vi "DiffDrivePoseEst2_Execute.vi"(0 "Vision TImeStamp_Seconds":dbl=0.02, 3 "DiffPoseEst2Config":T1={"TrackWidth_Meters"=1.2, "Odom X std dev M"=0.02, "Odom Y std dev M"=0.02, "Odom Heading std dev Rad"=0.01, "Vision X std dev M"=0.1, "Vision Y std dev M"=0.1, "Vision Heading std dev Rad"=0.05} {"Vision Heading std dev Rad" format="%#_13g"; "Vision Y std dev M" format="%#_13g"; "Vision X std dev M" format="%#_13g"; "Odom Heading std dev Rad" format="%#_13g"; "Odom Y std dev M" format="%#_13g"; "Odom X std dev M" format="%#_13g"; "TrackWidth_Meters" format="%#_13g"}, 4 "visionRobotPose":T2={"TRANSLATION"={"X"=0.0, "Y"=0.0}, "ROTATION"={"VALUE"=0.0, "COS"=1.0, "SIN"=0.0}} {"ROTATION"."SIN" format="%13.4f"; "ROTATION"."COS" format="%13.4f"; "ROTATION"."VALUE" format="%13.4f"; "TRANSLATION"."Y" format="%14.3f"; "TRANSLATION"."X" format="%14.3f"}, 5 "Game Started":bool=TRUE, 6 "Add Vision Meas":bool, 7 "InitialPose":T2={"TRANSLATION"={"X"=0.0, "Y"=0.0}, "ROTATION"={"VALUE"=0.0, "COS"=1.0, "SIN"=0.0}} {"ROTATION"."SIN" format="%13.4f"; "ROTATION"."COS" format="%13.4f"; "ROTATION"."VALUE" format="%13.4f"; "TRANSLATION"."Y" format="%14.3f"; "TRANSLATION"."X" format="%14.3f"}, 8 "Pass Through Time":dbl=-1.0, 9 "Gyro Degrees":dbl, 10 "RightDistance_M":dbl=0.02, 11 "LeftDistance_M":dbl=0.02) -> (1 "Error":bool, 2 "Estimated Pose":T2={"TRANSLATION"={"X"=0.0, "Y"=0.0}, "ROTATION"={"VALUE"=0.0, "COS"=1.0, "SIN"=0.0}} {"ROTATION"."SIN" format="%13.4f"; "ROTATION"."COS" format="%13.4f"; "ROTATION"."VALUE" format="%13.4f"; "TRANSLATION"."Y" format="%14.3f"; "TRANSLATION"."X" format="%14.3f"})   [LabVIEW 2019, in "Trajectory_Library.lvlib"]
doc: "This single call LabVIEW function wraps Differential Drive Odometry to fuse latency-compensated vision measurements with differential drive encoder measurements. It is intended to be a drop-in replacement for DiffDrvOdom2; in fact, if you never call DiffDrvPoseEst2_AddVisionMeasurement and only call DiffDrvPoseEst2_Update then this will behave exactly the same as DiffDrvOdom2.\n \nThis function should be called every robot loop, or perhaps put into a separaate loop.\n\nWhen the \"Game Started\" input is false, the position is reset using the initial pose, wheel distances, and gyro position. Use this to wait processing changes in measurements until the game starts.\n\nWhen a new vision measurement is available it can be passed into this function to merge it with the other odometry data. This is done by setting the \"Add Vision Meas\" input to TRUE. To promote stability of the pose estimate and make it robust to bad vision data, we recommend only adding vision measurements that are already within one meter or so of the current pose estimate.\n\nThe default standard deviations of the model states are 0.02 meters for x, 0.02 meters for y, and 0.01 radians for heading. The default standard deviations of the vision measurements are 0.1 meters for x, 0.1 meters for y, and 0.1 radians for heading.\n\nInputs: \n - DiffPoseEst2Config -- cluster -- Packed configuration data used to define how this function operates. It includes inforation used to define kinematics and position standard deviations.\n - Game Started -- boolean -- When FALSE, resets the initial position. (Default: TRUE)\n - InitialPose -- Pose2d -- Initial position. (meters, meters, rotation2d)\n - leftDistanceMeters -- double -- The distance traveled by the left encoder. (Meters)\n - rightDistanceMeters -- double -- The distance traveled by the right encoder. (Meters)\n - gyroAngle -- Rotation2d -- The current gyro angle. (Degrees)\n - Pass Through Time -- double -- Current FPGA time. If input is unwired, FPGA time will be read internally.\n - AddVisionMeas -- boolean -- When TRUE the provided vision measurement is merged with the odometry data.\n - VisionRobotPose -- Pose2d -- The pose from vision measurements.\n - Vision Time Stamp -- double -- The FPGA time stamp of the vision meausrement. This helps to account for latency of the vision measurement.\n \nOutputs:\n - EstimatedPose -- Pose2d -- Current estimated pose (meters, rotation2d) \n - Error -- boolean -- If TRUE, and error occured."
uses:
  Trajectory_Library.lvlib
  TypeDef/POSE2D.ctl
  TypeDef/TRANSLATION2D.ctl
  TypeDef/ROTATION2D.ctl
  TypeDef/DIFF_DRIVE_POSE_EST2_CONFIG.ctl
  Conv_Deg_Radians.vi
  Rotation2d_CreateAngle.vi
  Util_GetTime_U32.vi
  MatBuilder_Create.vi
  <vilib>/Rock Robotics/SystemInterfaces/NetworkCommunication/NetComm_UsageReport_report.vi
  DiffDrvOdom2_Reset.vi
  TimeInterpVariant_Clear.vi
  Pose2d_getRotation.vi
  Rotation2d_Minus.vi
  Rotation2d_UnaryMinus.vi
  Rotation2d_RotateBy.vi
  Rotation2d_CreateXY.vi
  Util_CalcDist.vi
  Util_GetTime_U64.vi
  Globals/Util_LibraryGlobals.vi
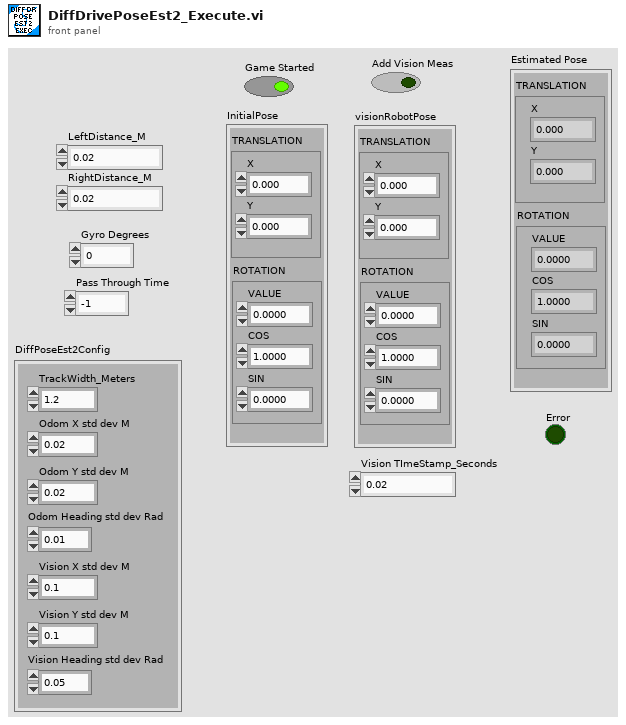
[diagram p1: front panel]
types:
  T1 = typedef "Trajectory_Library.lvlib/DIFF_DRIVE_POSE_EST2_CONFIG.ctl" = cluster{"TrackWidth_Meters":dbl, "Odom X std dev M":dbl, "Odom Y std dev M":dbl, "Odom Heading std dev Rad":dbl, "Vision X std dev M":dbl, "Vision Y std dev M":dbl, "Vision Heading std dev Rad":dbl}
  T2 = typedef "Trajectory_Library.lvlib/POSE2D.ctl" = cluster{"TRANSLATION":T3, "ROTATION":T4}
  T3 = typedef "Trajectory_Library.lvlib/TRANSLATION2D.ctl" = cluster{"X":dbl, "Y":dbl}
  T4 = typedef "Trajectory_Library.lvlib/ROTATION2D.ctl" = cluster{"VALUE":dbl, "COS":dbl, "SIN":dbl}
  T5 = typedef "NI_Matrix.lvlib/RealMatrix.ctl" = dbl[][]
  T6 = typedef "Trajectory_Library.lvlib/DIFF_DRIVE_KINEMATICS.ctl" = cluster{"TrackWidth_Meters":dbl}
  T7 = typedef "Trajectory_Library.lvlib/DIFF_DRIVE_POSE_EST2.ctl" = cluster{"M_Vision_K":T5, "m_nominal_dT":dbl, "m_PrevTime_Sec":dbl, "Pose_Buffer":T8, "Diff_Drive_Kinematics":T6, "Diff_Drive_Odom_2":T9, "M_Q":T5}
  T8 = typedef "Trajectory_Library.lvlib/TIME_INTERPOLATABLE_VARIANT.ctl" = cluster{"TimeStamps":dbl[], "DataArray":variant[], "Min_TimeStamp":dbl, "Max_TimeStamp":dbl, "ItemCount":i32, "MaxBufferTime":dbl}
  T9 = typedef "Trajectory_Library.lvlib/DIFF_DRIVE_ODOM2.ctl" = cluster{"M_POSE_Meters":T2, "M_GyroOffset":T4, "M_PrevAngle":T4, "M_PrevLeftDist_M":dbl, "M_PrevRightDist_M":dbl, "M_InitLeftDist_M":dbl, "M_InitRightDist_M":dbl}
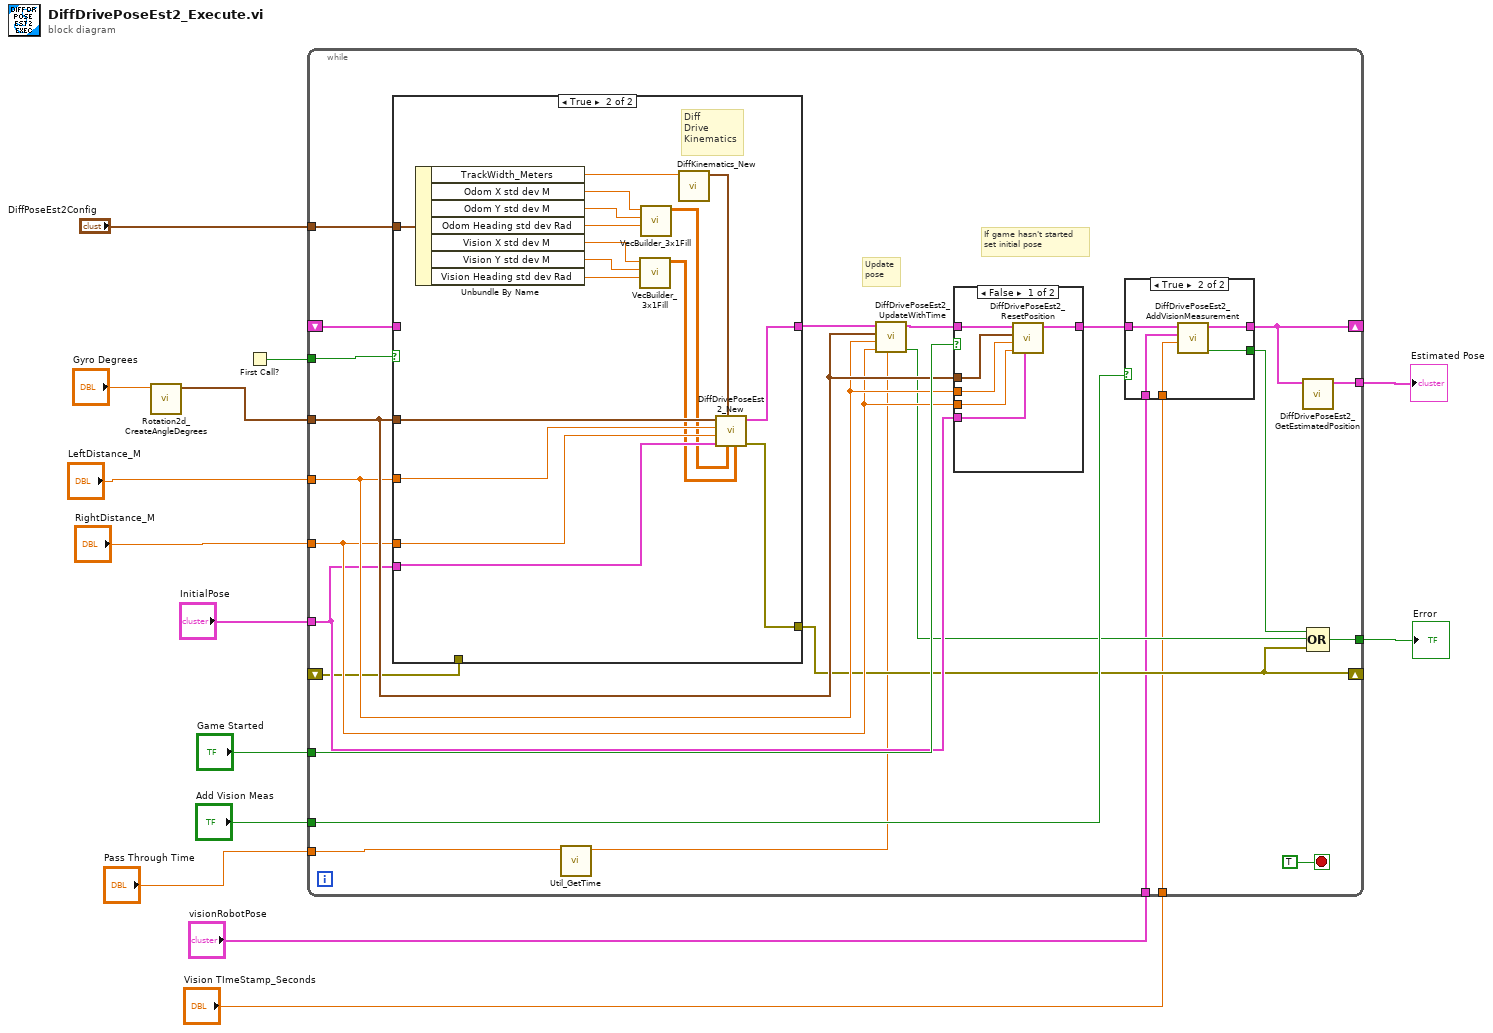
[diagram p0: block diagram]
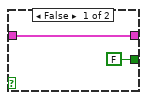
[diagram p3: hidden frame]
diagram:
  n1 = call "Rotation2d_CreateAngleDegrees.vi"("Angle_Degrees"="Gyro Degrees") -> ("ROTATION"=w3:T4)  [unwired: 10 in]
  n2 = First Call?() -> (First Call?: T/F=w14:bool)
  n3 = while {
    tunnel: w14 -> [w37]
    tunnel: w3 -> [w33]
    tunnel: "LeftDistance_M" -> [w32]
    tunnel: "RightDistance_M" -> [w31]
    tunnel: "InitialPose" -> [w30]
    tunnel: "Game Started" -> [w34]
    shift-right: [w23] -> _
    shift-left: _ -> [w28]
    tunnel: "Add Vision Meas" -> [w27]
    shift-right: [w24] -> _
    shift-left: _ -> [w18]
    tunnel: [w22] -> w8
    tunnel: [w21] -> w7
    tunnel: "visionRobotPose" -> [w20]
    tunnel: "Vision TImeStamp_Seconds" -> [w19]
    tunnel: "Pass Through Time" -> [w16]
    tunnel: "DiffPoseEst2Config" -> [w15]
    stop <- TRUE stop-if-true
    # "If game hasn't started\nset initial pose"
    # "Update\npose"
    n4 = case shown="True" w37 {
      tunnel: w33 -> [_ w70]
      tunnel: w32 -> [_ w69]
      tunnel: w31 -> [_ w68]
      tunnel: w30 -> [_ w67]
      tunnel: [w53 w66] -> w24
      tunnel: [w54 w65] -> w36
      tunnel: w28 -> [w54 _]
      tunnel: w18 -> [w53 _]
      tunnel: w15 -> [_ w64]
      frame False {
      }
      frame True {
        # "Diff\nDrive\nKinematics"
        n5 = Unbundle By Name(w64) -> ("TrackWidth_Meters"=w63:dbl, "Odom X std dev M"=w62:dbl, "Odom Y std dev M"=w61:dbl, "Odom Heading std dev Rad"=w60:dbl, "Vision X std dev M"=w59:dbl, "Vision Y std dev M"=w58:dbl, "Vision Heading std dev Rad"=w57:dbl)
        n6 = call "VecBuilder_3x1Fill.vi"("R2"=w57, "R1"=w58, "R0"=w59) -> ("output matrix"=w55:T5)  [unwired: 8 in]
        n7 = call "VecBuilder_3x1Fill.vi"("R2"=w60, "R1"=w61, "R0"=w62) -> ("output matrix"=w56:T5)  [unwired: 8 in]
        n8 = call "DiffKinematics_New.vi"("TrackWidth_Meters"=w63) -> ("DIFF_DRIVE_KINEMATICS"=w71:T6)  [unwired: 10 in]
        n9 = call "DiffDrivePoseEst2_New.vi"("VisionMeasurementStdDevs"=w55, "StateStdDevs"=w56, "DIFF_DRIVE_KINEMATICS"=w71, "InitialPose"=w67, "RightDistance_M"=w68, "LeftDistance_M"=w69, "gyroAngle"=w70) -> ("Error"=w66:errorcluster, "DiffDrivePoseEstimate"=w65:T7)  [unwired: 3 in]
      }
    }
    n10 = call "Util_GetTime.vi"("Pass_Through_Time"=w16) -> ("FPGA_Time_Seconds"=w17:dbl)  [unwired: 8 in, 2 out]
    n11 = call "DiffDrivePoseEst2_UpdateWithTime.vi"("CurrentTimeSeconds"=w17, "RightDistance"=w31, "LeftDistance"=w32, "GyroAngle"=w33, "in DiffDrivePoseEst2"=w36) -> ("Error"=w26:bool, "Out DiffDrivePoseEst2"=w35:T7)  [unwired: 4 in, 1 out]
    n12 = case shown="False" w34 {
      tunnel: w35 -> [w44 w45]
      tunnel: w33 -> [w43 _]
      tunnel: w32 -> [w42 _]
      tunnel: w31 -> [w41 _]
      tunnel: w30 -> [w40 _]
      tunnel: [w39 w45] -> w29
      frame False {
        n13 = call "DiffDrivePoseEst2_ResetPosition.vi"("Pose"=w40, "RightDistance_M"=w41, "LeftDistance_M"=w42, "Gyro"=w43, "in DiffDrivePoseEst2"=w44) -> ("Out DiffDrivePoseEst2"=w39:T7)  [unwired: 6 in]
      }
      frame True {
      }
    }
    n14 = case shown="True" w27 {
      tunnel: w29 -> [w47 w52]
      tunnel: [w47 w51] -> w23
      tunnel: [FALSE ("Error") w50] -> w25
      tunnel: w20 -> [_ w49]
      tunnel: w19 -> [_ w48]
      frame False {
      }
      frame True {
        n15 = call "DiffDrivePoseEst2_AddVisionMeasurement.vi"("TImeStamp_Seconds"=w48, "visionRobotPose"=w49, "in DiffDrivePoseEst2"=w52) -> ("Error"=w50:bool, "Out DiffDrivePoseEst2"=w51:T7)  [unwired: 7 in]
      }
    }
    n16 = call "DiffDrivePoseEst2_GetEstimatedPosition.vi"("in DiffDrivePoseEstimate"=w23) -> ("Estimated Pose"=w22:T2)  [unwired: 10 in]
    n17 = Compound Arithmetic op=OR(w25, w26, w24) -> (w21:bool)
  }
  "Estimated Pose" <- w8
  "Error" <- w7
